vi "PECD_V1.vi"() -> ()   [LabVIEW 2019]
uses:
  <vilib>/vision/NI_Vision_Development_Module.lvlib
panel:
  in  "Boolean":bool
  in  "?":refnum<k7>(container)
  in  "?":enum32{"Align", "Acquire"}(tab)
  in  "Mask Width":dbl
  in  "Threshold":dbl
  in  "Centroiding":bool
  in  "Accumulate":bool
  out "y_sum":cluster{dbl[], dbl[]}(graph)
  out "x_sum":cluster{dbl[], dbl[]}(graph)
  in  "y0 :":dbl=13.0
  in  "x0":dbl=-22.0
  out "Waveform Graph 2":dbl[](graph)
  out "Live Test View":dbl[][](graph)
  in  "?":bool
  out "Cropped Image":dbl[][](graph)
  in  "?":refnum<k7>(container)
  out "PECD":dbl[][](graph)
  in  "New Save After X Scans :":i32=1
  in  "Molecule :":string="R_Camphor"
  out "of":dbl
  out "Scan :":dbl
  out "of":dbl
  out "Scan :":dbl
  out "?":dbl[](graph)
  in  "No. of Photons :":dbl=3.0
  out "Waveform Graph 4":dbl[](graph)
  out "'On-the-fly' Legendre Polynomial Fit Coefficients":cluster{dbl[], dbl[]}(graph)
  out "RCP Angular Distribution":dbl[][](graph)
  out "LCP Angular Distribution":dbl[][](graph)
  in  "Centroiding :":bool
  out "LCP Signal":dbl[](graph)
  in  "LCP Position :":sgl=47.0
  in  "RCP Position :":sgl=137.0
  in  "No. of PECD Scans :":i32=10
  in  "Frames per Scan :":i32=50
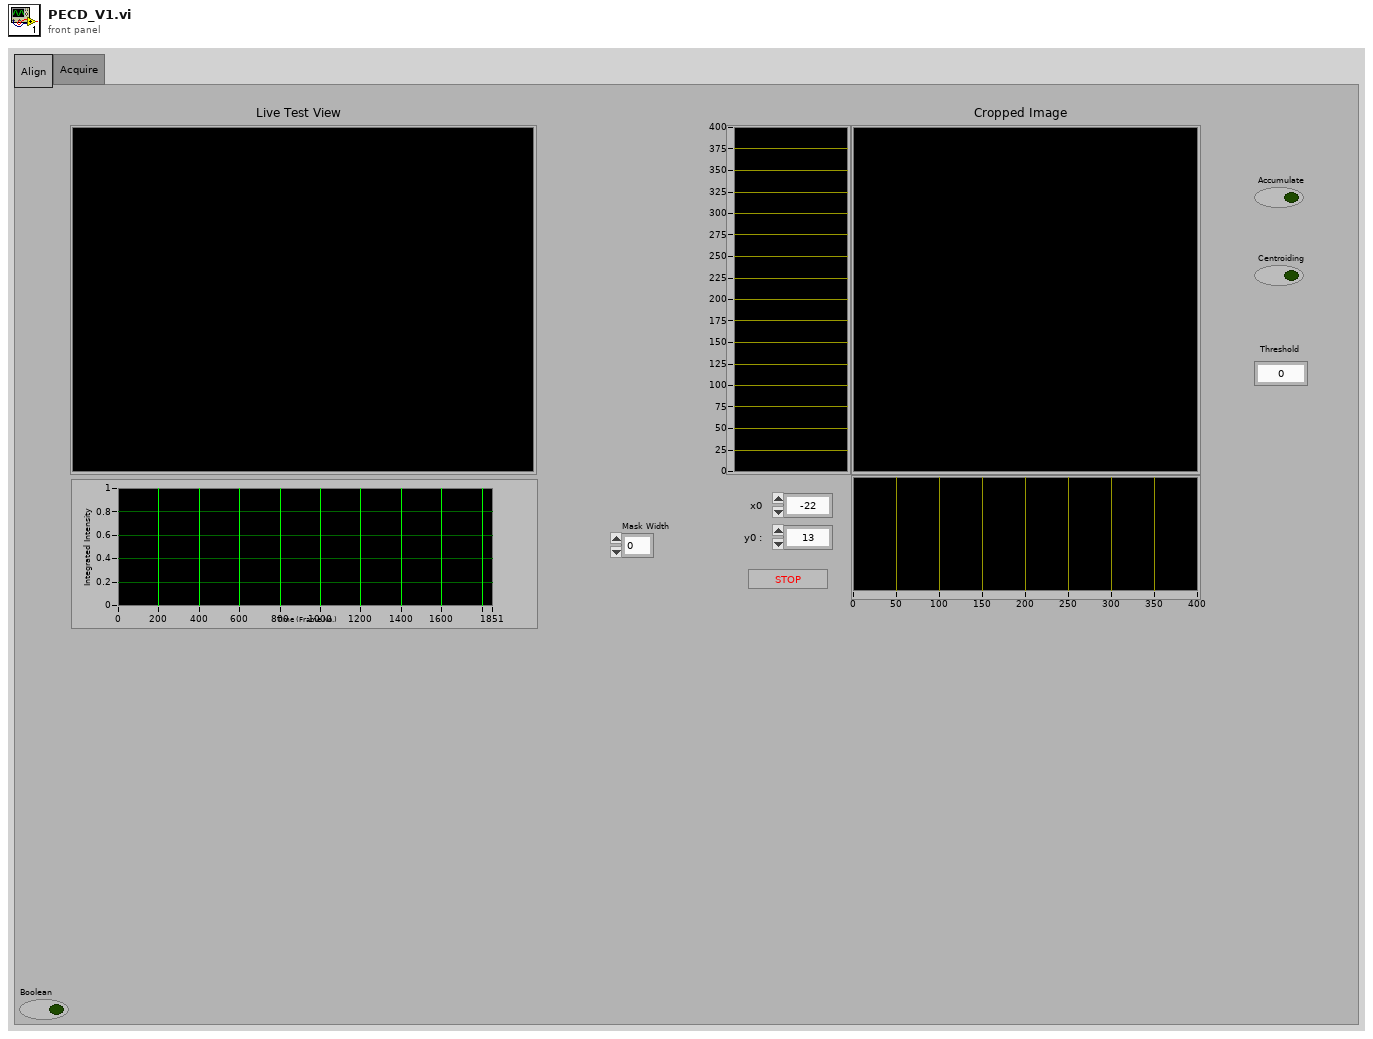
[diagram p1: front panel]
types:
  T1 = typedef "Image Type" = u32
  T2 = typedef "IMAQ Image.ctl" = refnum<image>
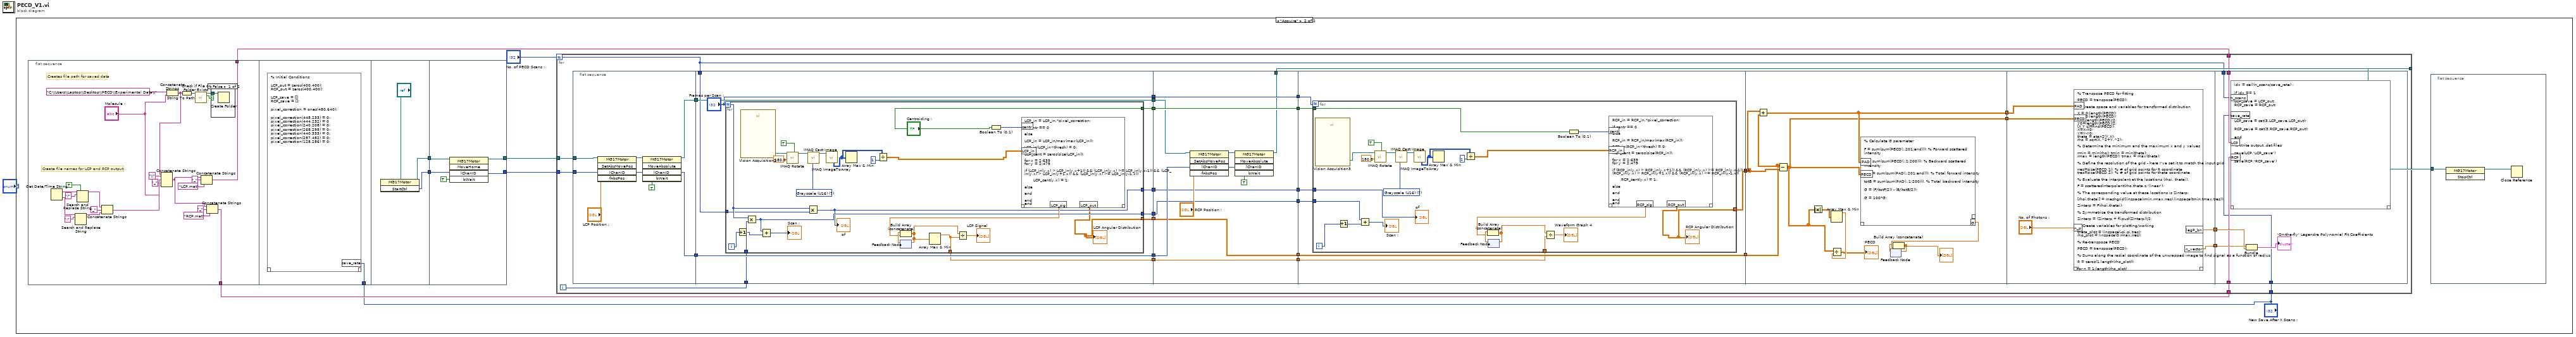
[diagram p0: block diagram]
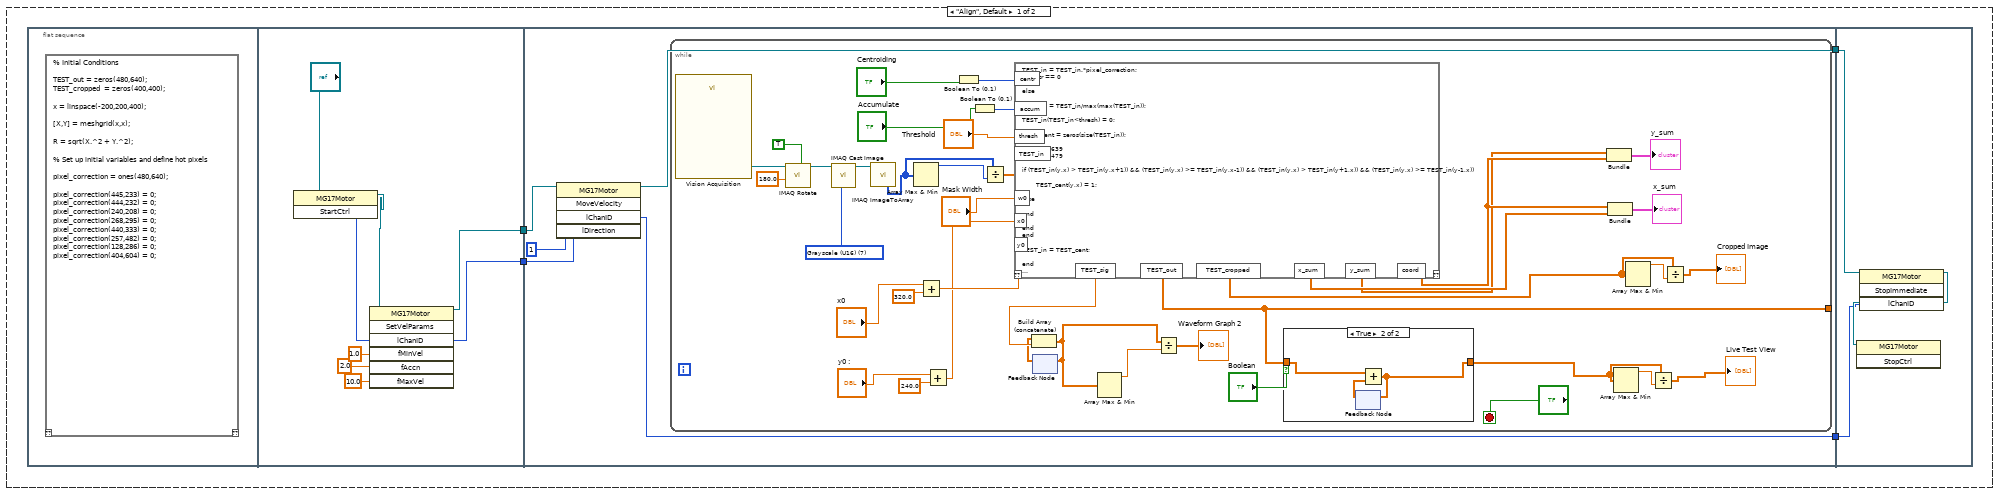
[diagram p2: hidden frame]
diagram:
  n1 = case shown="\"Acquire\"" "?" {
    frame "Align", Default {
      n2 = flat-sequence {
        tunnel: [w7] -> w5
        tunnel: [w6] -> w4
        tunnel: w5 -> [w17]
        tunnel: w4 -> [w16]
        tunnel: [w15] -> w3
        tunnel: [w14] -> w2
        tunnel: w3 -> [w65]
        tunnel: w2 -> [w63]
        frame #0 {
          n3 = script code="% Initial Conditions\n\nTEST_out = zeros(480,640);\nTEST_cropped  = zeros(400,400);\n\nx = linspace(-200,200,400);\n\n[X,Y] = meshgrid(x,x);\n\nR = sqrt(X.^2 + Y.^2);\n\n% Set up initial variables and define hot pixels\n\npixel_correction = ones(480,640);\n\npixel_correction(445,233) = 0;\npixel_correction(444,232) = 0;\npixel_correction(240,208) = 0;\npixel_correction(268,295) = 0;\npixel_correction(440,333) = 0;\npixel_correction(257,482) = 0;\npixel_correction(128,286) = 0;\npixel_correction(404,604) = 0;"() -> ()  [unwired: 1 in, 1 out]
        }
        frame #1 {
          n4 = invoke class="MG17Motor" method="StartCtrl"(reference="?") -> (reference out=w12:refnum<k7>, "StartCtrl"=w11:i32)  [unwired: 2 in, 1 out]
          n5 = invoke class="MG17Motor" method="SetVelParams"(reference=w12, "lChanID"=w11, "fMinVel"=sgl 1.0, "fAccn"=sgl 2.0, "fMaxVel"=sgl 10.0) -> (reference out=w7:refnum<k7>, "lChanID"=w6:i32)  [unwired: 2 in, 5 out]
        }
        frame #2 {
          n6 = invoke class="MG17Motor" method="MoveVelocity"(reference=w17, "lChanID"=w16, "lDirection"=1 ("lJogDir")) -> (reference out=w15:refnum<k7>, "lChanID"=w14:i32)  [unwired: 2 in, 3 out]
          n7 = while {
            tunnel: [w31] -> _
            stop <- "?" stop-if-true
            w58 = T1 7 items=["Grayscale (U8)", "Grayscale (I16)", "Grayscale (SGL)", "Complex (CSG)", "RGB (U32)", "HSL (U32)", "RGB (U64)", "Grayscale (U16)"] ("Image Type")
            n8 = call "Vision Acquisition"() -> ("Image Out"=w54:T2)  [unwired: 26 in, 1 out]
            n9 = call "IMAQ Rotate"("Maintain Size"=TRUE, "Angle (degrees)"=sgl 180.0, "Image Src"=w54) -> ("Image Dst Out"=w55:T2)  [unwired: 7 in, 1 out]
            n10 = call "IMAQ Cast Image"("Image Type"=w58, "Image Src"=w55) -> ("Image Dst Out"=w57:T2)  [unwired: 8 in, 1 out]
            n11 = call "IMAQ ImageToArray"("Image"=w57) -> ("Image Pixels (U16)"=w56:u16[][])  [unwired: 3 in, 4 out]
            n12 = Array Max & Min(array=w56) -> (max value=w33:u16)  [unwired: 3 out]
            n13 = Add(x="x0", y=320.0) -> (x+y=w40:dbl)
            n14 = Add(x="y0 :", y=240.0) -> (x+y=w39:dbl)
            n15 = Boolean To (0,1)(Boolean="Centroiding") -> (0, 1=w21:i16)
            n16 = Boolean To (0,1)(Boolean="Accumulate") -> (0, 1=w30:i16)
            n17 = Divide(x=w56, y=w33) -> (x/y=w51:dbl[][])
            n18 = script code="TEST_in = TEST_in.*pixel_correction;\nif centr == 0\n\nelse\n\nTEST_in = TEST_in/max(max(TEST_in));\n\nTEST_in(TEST_in<thresh) = 0;\n\nTEST_cent = zeros(size(TEST_in));\n\nfor x = 2:639\nfor y = 2:479\n\nif (TEST_in(y,x) > TEST_in(y,x+1)) && (TEST_in(y,x) >= TEST_in(y,x-1)) && (TEST_in(y,x) > TEST_in(y+1,x)) && (TEST_in(y,x) >= TEST_in(y-1,x))\n\n       TEST_cent(y,x) = 1;\n\nelse\n\nend\n\nend\nend\n\nTEST_in = TEST_cent;\n\nend\n\nif accum == 0\n\n     TEST_cropped = zeros(400,400);\n\n     TEST_out = zeros(480,640);\n\nelse\n\nend\n\nTEST_out = TEST_in;\n\nTEST_sig = sum(sum(TEST_out)); \n\nx_up = x0 + 200;\ny_up = y0 + 200;\nx_low = x0- 199;\ny_low = y0 - 199;\n\nTEST_cropped = TEST_out(x_low:x_up,y_low:y_up) + TEST_cropped;\n\nTEST_cropped = TEST_cropped.*(R>w0);\n\n\nx_sum = sum(TEST_cropped,1);\nx_sum = x_sum/max(x_sum);\n\ny_sum = sum(TEST_cropped,2);\ny_sum = y_sum'/max(y_sum);\n\ncoord = 1:400;"("TEST_in"=w51, "x0"=w39, "y0"=w40, "accum"=w30, "centr"=w21, "thresh"="Threshold", "w0"="Mask Width") -> ("TEST_out"=w31:dbl[][], "TEST_sig"=w49:dbl, "TEST_cropped"=w26:dbl[][], "x_sum"=w36:dbl[], "coord"=w35:dbl[], "y_sum"=w34:dbl[])  [unwired: 1 in, 1 out]
            n19 = feedback #1() -> (w45:dbl[])  [unwired: 1 in]
            n20 = Build Array (concatenate)(w45, w49) -> (w46:dbl[])
            n21 = feedback-in #1(w46) -> ()
            n22 = Array Max & Min(array=w46) -> (max value=w47:dbl)  [unwired: 3 out]
            n23 = Divide(x=w46, y=w47) -> (x/y=→"Waveform Graph 2":dbl[])
            n24 = case shown="True" "Boolean" {
              tunnel: w31 -> [w59 w61]
              tunnel: [w59 w60] -> w24
              frame False {
              }
              frame True {
                n25 = feedback #2() -> (w62:dbl[][])  [unwired: 1 in]
                n26 = Add(x=w61, y=w62) -> (x+y=w60:dbl[][])
                n27 = feedback-in #2(w60) -> ()
              }
            }
            n28 = Bundle(w34, w35) -> (→"y_sum":cluster{dbl[], dbl[]})  [unwired: 1 in]
            n29 = Bundle(w35, w36) -> (→"x_sum":cluster{dbl[], dbl[]})  [unwired: 1 in]
            n30 = Array Max & Min(array=w24) -> (max value=w25:dbl)  [unwired: 3 out]
            n31 = Array Max & Min(array=w26) -> (max value=w27:dbl)  [unwired: 3 out]
            n32 = Divide(x=w24, y=w25) -> (x/y=→"Live Test View":dbl[][])
            n33 = Divide(x=w26, y=w27) -> (x/y=→"Cropped Image":dbl[][])
          }
        }
        frame #3 {
          n34 = invoke class="MG17Motor" method="StopImmediate"(reference=w65, "lChanID"=w63) -> (reference out=w64:refnum<k7>)  [unwired: 2 in, 3 out]
          n35 = invoke class="MG17Motor" method="StopCtrl"(reference=w64) -> ()  [unwired: 2 in, 3 out]
        }
      }
    }
    frame "Acquire" {
      n36 = flat-sequence {
        tunnel: [w78] -> w68
        tunnel: [w77] -> w67
        tunnel: "New Save After X Scans :" -> [w102]
        tunnel: [w104] -> w70
        tunnel: [w103] -> w69
        tunnel: [w109] -> w71
        tunnel: [w106] -> w72
        tunnel: w70 -> [w108]
        tunnel: w69 -> [w110]
        frame #0 {
          # "Create file names for LCP and RCP output"
          # "Creates file path for saved data"
          n37 = Get Date/Time String() -> (date string=w96:string, time string=w93:string)  [unwired: 3 in]
          n38 = Search and Replace String(input string=w93, search string=":") -> (result string=w90:string)  [unwired: 6 in, 3 out]
          n39 = Search and Replace String(replace all?=TRUE ("replace all? (F)"), input string=w96, search string="/") -> (result string=w91:string)  [unwired: 5 in, 3 out]
          n40 = Concatenate Strings(w91, "_" ("string"), w90) -> (w88:string)
          n41 = Concatenate Strings("C:\\Users\\Laptop\\Desktop\\PECD\\Experimental Data\\", "Molecule :") -> (w80:string)
          n42 = Concatenate Strings(w80, "\\" ("string"), w88, "_" ("string"), "Molecule :") -> (w83:string)
          n43 = String To Path(string=w80) -> (path=w99:path)
          n44 = call <vilib>:"Check if File or Folder Exists.vi"("path"=w99) -> ("file or folder exists?"=w98:bool, "dup path"=w97:path)  [unwired: 8 in, 1 out]
          n45 = Concatenate Strings(w83, "_" ("string"), "LCP.mat" ("string")) -> (w78:string)
          n46 = Concatenate Strings(w83, "_" ("string"), "RCP.mat" ("string")) -> (w77:string)
          n47 = case shown="False" w98 {
            tunnel: w97 -> [w101 _]
            frame False {
              n48 = Create Folder(path (use dialog)=w101) -> ()  [unwired: 2 in, 3 out]
            }
            frame True {
            }
          }
        }
        frame #1 {
          n49 = script code="% Initial Conditions\n\nLCP_out = zeros(400,400);\nRCP_out = zeros(400,400);\n\nLCP_save = [];\nRCP_save = [];\n\npixel_correction = ones(480,640);\n\npixel_correction(445,233) = 0;\npixel_correction(444,232) = 0\npixel_correction(240,208) = 0;\npixel_correction(268,295) = 0;\npixel_correction(440,333) = 0;\npixel_correction(257,482) = 0;\npixel_correction(128,286) = 0;"("save_rate"=w102) -> ()  [unwired: 1 in, 1 out]
        }
        frame #2 {
          n50 = invoke class="MG17Motor" method="StartCtrl"(reference="?") -> (reference out=w103:refnum<k7>, "StartCtrl"=w104:i32)  [unwired: 2 in, 1 out]
        }
        frame #3 {
          n51 = invoke class="MG17Motor" method="MoveHome"(reference=w110, "lChanID"=w108, "bWait"=TRUE) -> (reference out=w109:refnum<k7>, "lChanID"=w106:i32)  [unwired: 2 in, 3 out]
        }
      }
      n52 = for {
        N: "No. of PECD Scans :" -> [w112]
        tunnel: w71 -> [w138]
        tunnel: w72 -> [w137]
        tunnel: [w120] -> w73
        tunnel: w68 -> [w114]
        tunnel: w67 -> [w113]
        tunnel: "New Save After X Scans :" -> [w111]
        i -> [w119]
        n53 = flat-sequence {
          tunnel: w138 -> [w148]
          tunnel: w137 -> [w147]
          tunnel: [w142] -> w135
          tunnel: [w141] -> w133
          tunnel: [w158] -> w140
          tunnel: [w157] -> w136
          tunnel: w135 -> [w157]
          tunnel: [w156] -> w134
          tunnel: w133 -> [w156]
          tunnel: [w155] -> w129
          tunnel: ["Frames per Scan :"] -> w126
          tunnel: [w153] -> w123
          tunnel: w119 -> [w152]
          tunnel: w112 -> [w151]
          tunnel: [w150] -> w118
          tunnel: [w149] -> w115
          tunnel: w140 -> [w196]
          tunnel: [w196] -> w139
          tunnel: w136 -> [w191]
          tunnel: w134 -> [w190]
          tunnel: [w189] -> w130
          tunnel: w129 -> [w189]
          tunnel: w126 -> [w188]
          tunnel: [w188] -> w125
          tunnel: [w187] -> w124
          tunnel: w123 -> [w187]
          tunnel: [w186] -> w120
          tunnel: w118 -> [w185]
          tunnel: [w185] -> w117
          tunnel: [w184] -> w116
          tunnel: w115 -> [w184]
          tunnel: w139 -> [w203]
          tunnel: [w200] -> w132
          tunnel: [w202] -> w131
          tunnel: w130 -> [w202]
          tunnel: w125 -> [w201]
          tunnel: w124 -> [w199]
          tunnel: w117 -> [w198]
          tunnel: w116 -> [w197]
          tunnel: w132 -> [w231]
          tunnel: w131 -> [w230]
          tunnel: [w228] -> w128
          tunnel: [w235] -> w127
          tunnel: w128 -> [w240]
          tunnel: w127 -> [w239]
          tunnel: [w237] -> w122
          tunnel: [w236] -> w121
          tunnel: w122 -> [w247]
          tunnel: w121 -> [w246]
          tunnel: w114 -> [w244]
          tunnel: w113 -> [w243]
          tunnel: w112 -> [w242]
          tunnel: w111 -> [w241]
          frame #0 {
            n54 = invoke class="MG17Motor" method="SetAbsMovePos"(reference=w148, "lChanID"=w147, "fAbsPos"="LCP Position :") -> (reference out=w145:refnum<k7>, "lChanID"=w144:i32)  [unwired: 2 in, 3 out]
            n55 = invoke class="MG17Motor" method="MoveAbsolute"(reference=w145, "lChanID"=w144, "bWait"=TRUE) -> (reference out=w142:refnum<k7>, "lChanID"=w141:i32)  [unwired: 2 in, 3 out]
          }
          frame #1 {
            n56 = for {
              N: "Frames per Scan :" -> [w170]
              tunnel: [w162] -> w155
              tunnel: ["Centroiding :"] -> w158
              tunnel: [w173] -> w153
              tunnel: w152 -> [w172]
              tunnel: w151 -> [w169]
              tunnel: [w166] -> w150
              tunnel: [w165] -> w149
              i -> [w167]
              w183 = T1 7 items=["Grayscale (U8)", "Grayscale (I16)", "Grayscale (SGL)", "Complex (CSG)", "RGB (U32)", "HSL (U32)", "RGB (U64)", "Grayscale (U16)"] ("Image Type")
              n57 = Increment(x=w167) -> (x+1=w168:i32)
              n58 = call "Vision Acquisition2"() -> ("Image Out"=w164:T2)  [unwired: 26 in, 1 out]
              n59 = Multiply(x=w170, y=w172) -> (x*y=w166:i32)
              n60 = Add(x=w166, y=w168) -> (x+y=→"Scan :":i32)
              n61 = call "IMAQ Rotate"("Maintain Size"=TRUE, "Angle (degrees)"=sgl 180.0, "Image Src"=w164) -> ("Image Dst Out"=w180:T2)  [unwired: 7 in, 1 out]
              n62 = Multiply(x=w170, y=w169) -> (x*y=w165:i32)
              "of" <- w165
              n63 = call "IMAQ Cast Image"("Image Type"=w183, "Image Src"=w180) -> ("Image Dst Out"=w182:T2)  [unwired: 8 in, 1 out]
              n64 = call "IMAQ ImageToArray"("Image"=w182) -> ("Image Pixels (U16)"=w181:u16[][])  [unwired: 3 in, 4 out]
              n65 = Array Max & Min(array=w181) -> ()  [unwired: 4 out]
              n66 = Divide(x=w181, y=1) -> (x/y=w161:dbl[][])
              n67 = feedback #3() -> (w176:dbl[])  [unwired: 1 in]
              n68 = Boolean To (0,1)(Boolean="Centroiding :") -> (0, 1=w160:i16)
              n69 = script code="LCP_in = LCP_in.*pixel_correction;\n\nif centr == 0\n\nelse\n\nLCP_in = LCP_in/max(max(LCP_in));\n\nLCP_in(LCP_in<thresh) = 0;\n\nLCP_cent = zeros(size(LCP_in));\n\nfor x = 2:639\nfor y = 2:479\n\nif (LCP_in(y,x) > LCP_in(y,x+1)) && (LCP_in(y,x) >= LCP_in(y,x-1)) && (LCP_in(y,x) > LCP_in(y+1,x)) && (LCP_in(y,x) >= LCP_in(y-1,x))\n\n       LCP_cent(y,x) = 1;\n\nelse\n\nend\n\nend\nend\n\nLCP_in = LCP_cent;\n\nend\n\nLCP_out = LCP_out + LCP_in(x_low:x_up,y_low:y_up);\n\nLCP_sig = sum(sum(LCP_in));"("LCP_in"=w161, "centr"=w160) -> ("LCP_out"=w162:dbl[][], "LCP_sig"=w175:dbl)  [unwired: 1 in, 1 out]
              "LCP Angular Distribution" <- w162
              n70 = Build Array (concatenate)(w176, w175) -> (w174:dbl[])
              n71 = feedback-in #3(w174) -> ()
              n72 = Array Max & Min(array=w174) -> (max value=w173:dbl)  [unwired: 3 out]
              n73 = Divide(x=w174, y=w173) -> (x/y=→"LCP Signal":dbl[])
            }
          }
          frame #2 {
            n74 = invoke class="MG17Motor" method="SetAbsMovePos"(reference=w191, "lChanID"=w190, "fAbsPos"="RCP Position :") -> (reference out=w194:refnum<k7>, "lChanID"=w193:i32)  [unwired: 2 in, 3 out]
            n75 = invoke class="MG17Motor" method="MoveAbsolute"(reference=w194, "lChanID"=w193, "bWait"=TRUE) -> (reference out=w186:refnum<k7>)  [unwired: 2 in, 4 out]
          }
          frame #3 {
            n76 = for {
              N: w201 -> [_]
              tunnel: w203 -> [w205]
              tunnel: [w207] -> w200
              tunnel: w199 -> [w215]
              tunnel: w198 -> [w212]
              tunnel: w197 -> [w210]
              i -> [w214]
              w225 = T1 7 items=["Grayscale (U8)", "Grayscale (I16)", "Grayscale (SGL)", "Complex (CSG)", "RGB (U32)", "HSL (U32)", "RGB (U64)", "Grayscale (U16)"] ("Image Type")
              n77 = call "Vision Acquisition3"() -> ("Image Out"=w209:T2)  [unwired: 26 in, 1 out]
              n78 = Increment(x=w214) -> (x+1=w213:i32)
              n79 = Add(x=w212, y=w213) -> (x+y=→"Scan :":i32)
              n80 = call "IMAQ Rotate"("Maintain Size"=TRUE, "Angle (degrees)"=sgl 180.0, "Image Src"=w209) -> ("Image Dst Out"=w222:T2)  [unwired: 7 in, 1 out]
              n81 = call "IMAQ Cast Image"("Image Type"=w225, "Image Src"=w222) -> ("Image Dst Out"=w224:T2)  [unwired: 8 in, 1 out]
              n82 = call "IMAQ ImageToArray"("Image"=w224) -> ("Image Pixels (U16)"=w223:u16[][])  [unwired: 3 in, 4 out]
              n83 = Array Max & Min(array=w223) -> ()  [unwired: 4 out]
              n84 = Divide(x=w223, y=1) -> (x/y=w204:dbl[][])
              n85 = feedback #4() -> (w217:dbl[])  [unwired: 1 in]
              n86 = Boolean To (0,1)(Boolean=w205) -> (0, 1=w206:i16)
              n87 = script code="RCP_in = RCP_in.*pixel_correction;\n\nif centr == 0\n\nelse\n\nRCP_in = RCP_in/max(max(RCP_in));\n\nRCP_in(RCP_in<thresh) = 0;\n\nRCP_cent = zeros(size(RCP_in));\n\nfor x = 2:639\nfor y = 2:479\n\nif (RCP_in(y,x) > RCP_in(y,x+1)) && (RCP_in(y,x) >= RCP_in(y,x-1)) && (RCP_in(y,x) > RCP_in(y+1,x)) && (RCP_in(y,x) >= RCP_in(y-1,x))\n\n       RCP_cent(y,x) = 1;\n\nelse\n\nend\n\nend\nend\n\nRCP_in = RCP_cent;\n\nend\n\nRCP_out = RCP_out + RCP_in(x_low:x_up,y_low:y_up);\n\nRCP_sig = sum(sum(RCP_in));"("RCP_in"=w204, "cent"=w206) -> ("RCP_out"=w207:dbl[][], "RCP_sig"=w216:dbl)  [unwired: 1 in, 1 out]
              "RCP Angular Distribution" <- w207
              n88 = Build Array (concatenate)(w217, w216) -> (w218:dbl[])
              n89 = feedback-in #4(w218) -> ()
              n90 = Divide(x=w218, y=w215) -> (x/y=→"Waveform Graph 4":dbl[])
              "of" <- w210
            }
          }
          frame #4 {
            n91 = Add(x=w231, y=w230) -> (x+y=w235:dbl[][])
            n92 = Subtract(x=w230, y=w231) -> (x-y=w228:dbl[][])
            n93 = Absolute Value(x=w228) -> (abs(x)=w229:dbl[][])
            n94 = Array Max & Min(array=w229) -> (max value=w227:dbl)  [unwired: 3 out]
            n95 = Divide(x=w228, y=w227) -> (x/y=→"PECD":dbl[][])
            n96 = script code="% Calculate G parameter\n\nF = sum(sum(PECD(:,201:end))); % Forward scattered intensity\n\nB = sum(sum(PECD(:,1:200))); % Backward scattered intensity\n\ntotF = sum(sum(PAD(:,201:end))); % Total forward intensity\n\ntotB = sum(sum(PAD(:,1:200))), % Total backward intensity\n\nG = (F/(totF/2)) - (B/(totB/2));\n\nG = 100*G;"("PAD"=w235, "PECD"=w228) -> ("G"=w234:dbl)  [unwired: 1 in, 1 out]
            n97 = feedback #5() -> (w233:dbl[])  [unwired: 1 in]
            n98 = Build Array (concatenate)(w233, w234) -> (w232:dbl[])
            "?" <- w232
            n99 = feedback-in #5(w232) -> ()
          }
          frame #5 {
            n100 = script code="% Transpose PECD for fitting\n\nPECD = transpose(PECD);\n\n% Create space and variables for transformed distribution\n\nX = 0:length(PECD);\nY = 0:length(PECD);\nX0=length(PECD)/2;\nY0=length(PECD)/2;\n[X Y z]=find(PECD);\nX=X-X0;\nY=Y-Y0;\ntheta = atan2(Y,X);\nrho = sqrt(X.^2+Y.^2);\n\n% Determine the minimum and the maximum x and y values\n\nrmin = min(rho); tmin = min(theta);\nrmax = length(PECD); tmax = max(theta);\n\n% Define the resolution of the grid - here I've set it to match the input grid\n\nrres=size(PECD,1); % # of grid points for R coordinate\ntres=size(PECD,2); % # of grid points for theta coordinate\n\n% Evaluate the interpolant at the locations (rhoi, thetai).\n\nF = scatteredInterpolant(rho,theta,z,'linear');\n\n% The corresponding value at these locations is Zinterp:\n\n[rhoi,thetai] = meshgrid(linspace(rmin,rmax,rres),linspace(tmin,tmax,tres));\n\nZinterp = F(rhoi,thetai);\n\n% Symmetrize the transformed distribution\n \nZinterp = (Zinterp + flipud(Zinterp))/2;\n\n% Create variables for plotting/working\n \ntheta_plot = linspace(-pi,pi,tres);\nrho_plot = linspace(0,rmax,rres);\n\n% Re-transpose PECD\n\nPECD = transpose(PECD);\n\n% Sums along the radial coordinate of the unwrapped image to find signal as a function of radius\n\nR = zeros(1,length(rho_plot));\n\nfor n = 1:length(rho_plot)\n    \n    f = abs(rho_plot(1,n)*(Zinterp(:,n))'.*sin(theta_plot));\n    \n    R(1,n) = sum(f);\n    \n    E(:,n) = rho_plot(1,n)*(Zinterp(:,n))';\n    \nend\n\nE = E/max(max(E));\n\nR = R/max(R);\n\nA = zeros(1,length(theta_plot));\n    \n% Finds the most prominent N peaks below R_cutoff\n\nR_cutoff = 200;\n\nN = 1;\n\n[val idx] = min(abs(rho_plot-R_cutoff));\n\ncutoff = idx;\n\n[val, idx, width] = findpeaks(R(1,1:cutoff),'NPeaks',N,'SortStr','descend','WidthReference','halfheight');\n\n% Finds the angular dependance of the PAD at the peaks\n\nfor n = 1:N\n    \n    a = mean(Zinterp(:,idx(1,n)-2:idx(1,n)+2),2);\n\n    A(n,:) = a;\n    \nend\n\n\n% Set up angular fit\n\n[xData, yData] = prepareCurveData( theta_plot, A );\n\nif n_p == 1\n    \n        ft = fittype( {'1', 'legendreP(1,cos(x))', 'legendreP(2,cos(x))'}, 'independent', 'x', 'dependent', 'y', 'coefficients', {'b0', 'b1', 'b2'} );\n        \n    elseif n_p == 2\n        \n        ft = fittype( {'1', 'legendreP(1,cos(x))', 'legendreP(2,cos(x))', 'legendreP(3,cos(x))', 'legendreP(4,cos(x))'}, 'independent', 'x', 'dependent', 'y', 'coefficients', {'b0', 'b1', 'b2', 'b3', 'b4'} );\n        \n    elseif n_p == 3\n        \n        ft = fittype( {'1', 'legendreP(1,cos(x))', 'legendreP(2,cos(x))', 'legendreP(3,cos(x))', 'legendreP(4,cos(x))', 'legendreP(5,cos(x))', 'legendreP(6,cos(x))'}, 'independent', 'x', 'dependent', 'y', 'coefficients', {'b0', 'b1', 'b2', 'b3', 'b4', 'b5', 'b6'} );\n        \n    elseif n_p == 4\n        \n        ft = fittype( {'1', 'legendreP(1,cos(x))', 'legendreP(2,cos(x))', 'legendreP(3,cos(x))', 'legendreP(4,cos(x))', 'legendreP(5,cos(x))', 'legendreP(6,cos(x))', 'legendreP(7,cos(x))', 'legendreP(8,cos(x))'}, 'independent', 'x', 'dependent', 'y', 'coefficients', {'b0', 'b1', 'b2', 'b3', 'b4', 'b5', 'b6', 'b7', 'b8'} );\n        \nend\n\n% Fit legendreP functions to the angular distribution\n\n[fitresult, gof] = fit( xData, yData, ft );\n\n% Extract fitting coefficients\n\nlegP_bn = coeffvalues(fitresult);\n\n     n_vector = [0:2*n_p];"("PECD"=w240, "PAD"=w239, "n_p"="No. of Photons :") -> ("legP_bn"=w236:dbl[], "n_vector"=w237:dbl[])  [unwired: 1 in, 1 out]
          }
          frame #6 {
            n101 = script code="idx = ceil(n_scans/save_rate) ;\n\nif idx == 1\n\nLCP_save = LCP_out;\nRCP_save = RCP_out;\n\nelse\n\nLCP_save = cat(3,LCP_save,LCP_out);\n\nRCP_save = cat(3,RCP_save,RCP_out);\n\nend\n\n% Write output .dat files\n\nsave(LCP,'LCP_save')\n\nsave(RCP,'RCP_save')"("LCP"=w244, "RCP"=w243, "n_scans"=w242, "save_rate"=w241) -> ()  [unwired: 1 in, 1 out]
            n102 = Bundle(w247, w246) -> (→"'On-the-fly' Legendre Polynomial Fit Coefficients":cluster{dbl[], dbl[]})  [unwired: 1 in]
          }
        }
      }
      n103 = flat-sequence {
        tunnel: w73 -> [w75]
        frame #0 {
          n104 = invoke class="MG17Motor" method="StopCtrl"(reference=w75) -> (reference out=w76:refnum<k7>)  [unwired: 2 in, 2 out]
          n105 = Close Reference(reference=w76) -> ()  [unwired: 1 in, 1 out]
        }
      }
    }
  }
